vi "Configure.vi"(0 "SG Path Power Meter Accessor in":refnum<class "SG Path Accessor.lvclass">, 5 "frequency":dbl=50000000.0, 11 "error in":errorcluster) -> (4 "SG Path Power Meter Accessor out":refnum<class "SG Path Accessor.lvclass">, 15 "error out":errorcluster)   [LabVIEW 2023, in "RS NRPx Power Meter.lvlib" / "SG Path Accessor.lvclass"]
uses:
  SG Path Accessor.lvclass
  Power Meter/Power Meter.lvclass
  Power Meter/Power Meter.lvclass/Power Meter.ctl
  Power Meter/Properties/Read Resource Name.vi
  SG Path Accessor.lvclass/SG Path Accessor.ctl
  Instruments/Power Meter/Power Meter Factory/Power Meter Factory.lvclass
  <instrlib>/Rohde&Schwarz Power Meter/Rohde&Schwarz Power Meter.lvlib
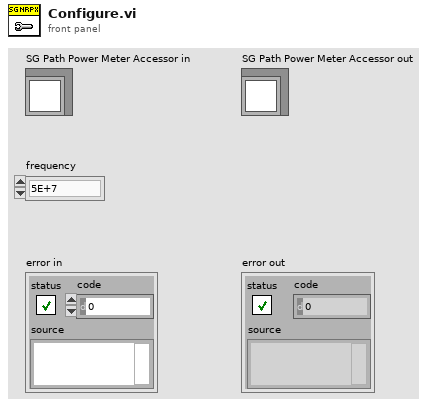
[diagram p1: front panel]
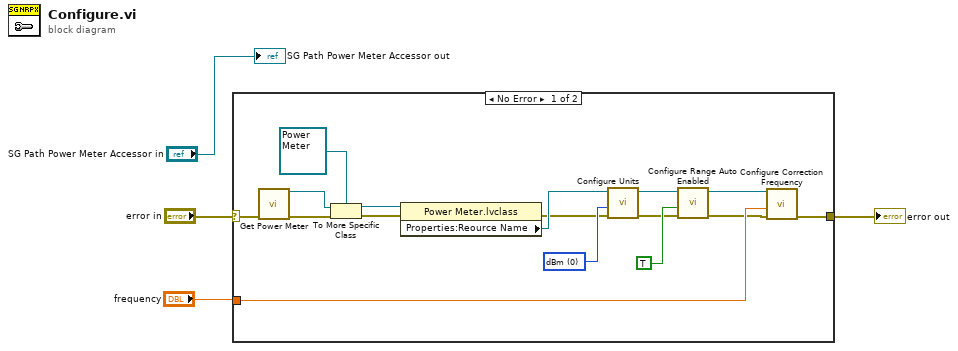
[diagram p0: block diagram]
diagram:
  n1 = case shown="No Error" "error in" {
    selector: "error in" -> [w20 w21]
    tunnel: [w9 w21] -> w4
    tunnel: "frequency" -> [w10 _]
    frame No Error {
      w14 = 0 items=["dBm", "W", "dBuv"] ("Units (dBm)")
      n2 = call "Get Power Meter.vi"("error in (no error)"=w20) -> ("Power Meter Base out"=w15:refnum<class "Power Meter Base.lvclass">, "error out"=w17:errorcluster)  [unwired: 13 in]
      n3 = To More Specific Class(target class=refnum<class "Power Meter.lvclass"> refnum ("PM NI568X in"), reference=w15, error in=w17) -> (specific class reference=w18:refnum<class "Power Meter.lvclass">, error out=w19:errorcluster)
      n4 = property class="Power Meter.lvclass"(reference=w18, error in=w19) -> (error out=w5:errorcluster, "Properties:Reource Name"=w6:refnum<visa-resource-name>)  [unwired: 1 out]
      n5 = call <instrlib>:"Configure Units.vi"("error in (no error)"=w5, "Units (dBm)"=w14, "VISA resource name"=w6) -> ("error out"=w11:errorcluster, "VISA resource name out"=w13:refnum<visa-resource-name>)  [unwired: 7 in]
      n6 = call <instrlib>:"Configure Range Auto Enabled.vi"("error in (no error)"=w11, "Range Auto Enabled (Off)"=TRUE, "VISA resource name"=w13) -> ("error out"=w8:errorcluster, "VISA resource name out"=w7:refnum<visa-resource-name>)  [unwired: 7 in]
      n7 = call <instrlib>:"Configure Correction Frequency.vi"("error in (no error)"=w8, "Correction Frequency (0Hz)"=w10, "VISA resource name"=w7) -> ("error out"=w9:errorcluster)  [unwired: 7 in, 1 out]
    }
    frame Error {
    }
  }
  "error out" <- w4
  "SG Path Power Meter Accessor out" <- "SG Path Power Meter Accessor in"
